vi "Convert Variant To Value.vi"(7 "姓名 in":string, 9 "error in":errorcluster, 10 "Value":variant) -> (1 "error out":errorcluster, 2 "姓名 out":string)   [LabVIEW 2015]
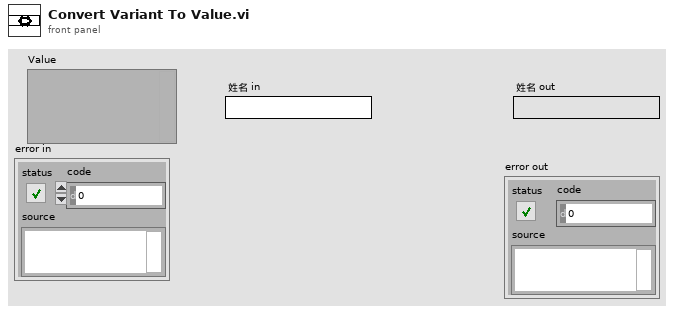
[diagram p1: front panel]
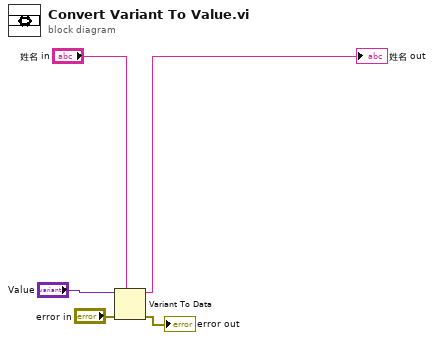
[diagram p0: block diagram]
diagram:
  n1 = Variant To Data(error in="error in", type="姓名 in", Variant="Value") -> (data=→"姓名 out":string, error out=→"error out":errorcluster)
